vi "Laurel Item Read.vi"(6 "Connection Type":T1, 7 "VISA resource name":refnum<visa-resource-name>, 8 "error in (no error)":errorcluster, 10 "byte count":i32=9, 11 "TCP Network Connection in":refnum<k5>) -> (0 "error out":errorcluster, 1 "trimmed string":string, 2 "Numeric":dbl, 3 "TCP Network Connection out":refnum<k5>, 5 "VISA resource name 2":refnum<visa-resource-name>)   [LabVIEW 2023]
uses:
  Type Definitions/Laurel Connection Type.ctl
  <vilib>/Utility/error.llb/whitespace.ctl
  <vilib>/Utility/error.llb/Trim Whitespace One-Sided.vi
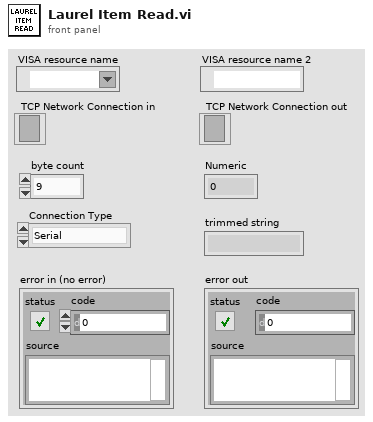
[diagram p1: front panel]
types:
  T1 = typedef "Laurel Connection Type.ctl" = enum16{"Serial", "TCP"}
  T2 = typedef "whitespace.ctl" = u16
  T3 = enum16{"Standard", "Buffered", "CRLF", "Immediate"}
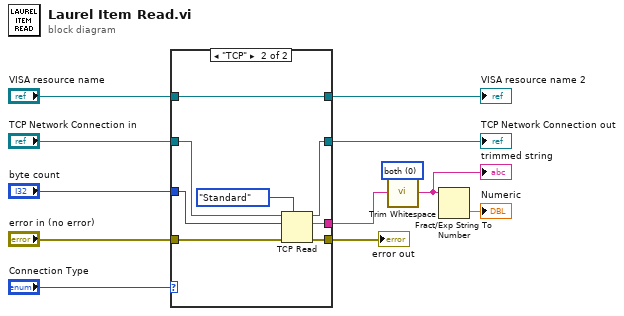
[diagram p0: block diagram]
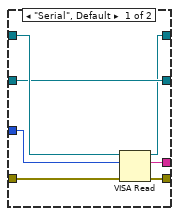
[diagram p2: hidden frame]
diagram:
  w6 = T2 0 items=["both", "start of string", "end of string"] ("location (both)")
  n1 = case shown="\"TCP\"" "Connection Type" {
    tunnel: [w15 w27] -> w12
    tunnel: [w17 w26] -> w11
    tunnel: [w16 w24] -> w10
    tunnel: "byte count" -> [w13 w23]
    tunnel: "error in (no error)" -> [w18 w22]
    tunnel: "TCP Network Connection in" -> [w15 w21]
    tunnel: "VISA resource name" -> [w19 w20]
    tunnel: [w14 w20] -> w1
    frame "Serial", Default {
      n2 = VISA Read(VISA resource name=w19, byte count=w13, error in (no error)=w18) -> (VISA resource name out=w14:refnum<visa-resource-name>, read buffer=w16:string, error out=w17:errorcluster)  [unwired: 1 out]
    }
    frame "TCP" {
      n3 = TCP Read(connection ID=w21, bytes to read=w23, error in (no error)=w22, 7:T3."Standard" ("mode (standard)")) -> (connection ID out=w27:refnum<k5>, data out=w24:string, error out=w26:errorcluster)  [unwired: 1 in]
    }
  }
  "TCP Network Connection out" <- w12
  "error out" <- w11
  "VISA resource name 2" <- w1
  n4 = call <vilib>:"Trim Whitespace.vi"("string"=w10, "location (both)"=w6) -> ("trimmed string"=w5:string)
  "trimmed string" <- w5
  n5 = Fract/Exp String To Number(string=w5) -> (number=→"Numeric":dbl)  [unwired: 3 in, 1 out]
